vi "Power Measurement Test.vi"(8 "error in (no error)":errorcluster, 9 "Power Measurements":string[](array[string]), 10 "Position":u32, 11 "Measurement in":refnum<class "Measurement.lvclass">) -> (0 "error out":errorcluster, 3 "Passed":bool)   [LabVIEW 2015, in "Measurement.lvclass"]
uses:
  Measurement.lvclass
  Driver Test/Measurement Type -- Enum.ctl
  <vilib>/regexp/Match Regular Expression.xnode
  Driver Test/Driver Test.lvclass
  Test Class/Test Class.lvclass
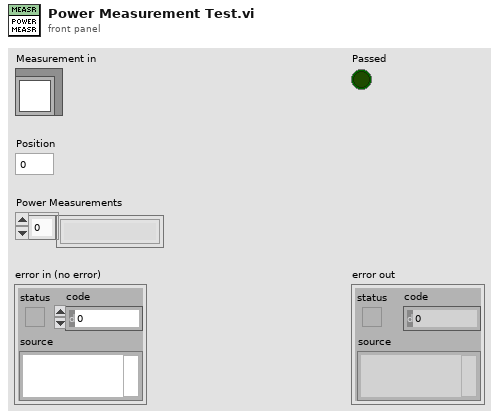
[diagram p1: front panel]
types:
  T1 = typedef "Driver Test.lvclass/Measurement Type -- Enum.ctl" = enum16{"DPM", "DAQmx", "ACPS Voltage", "ACPS Current", "ACPS Power", "DCPS Voltage", "DCPS Current", "DCPS Power"}
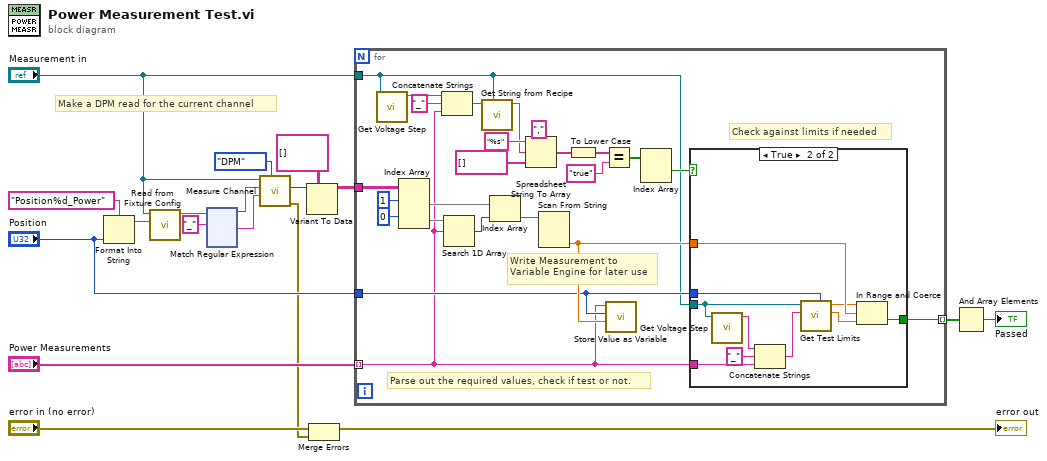
[diagram p0: block diagram]
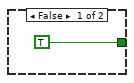
[diagram p2: hidden frame]
diagram:
  # "Make a DPM read for the current channel"
  n1 = Format Into String(format string="Position%d_Power", "Position") -> (resulting string=w16:string)  [unwired: 2 in, 1 out]
  n2 = call-dynamic "Read from Fixture Config.vi"("Key"=w16, "Test Class in"="Measurement in") -> ("Instrument Info"=w13:string)  [unwired: 8 in, 1 out]
  n3 = xnode "Match Regular Expression"("input string"=w13, "regular expression"="_") -> ("before match"=w12:string, "after match"=w11:string)  [unwired: 4 in, 3 out]
  n4 = call "Measure Channel.vi"("Measurement Type"=Measurement_Type_--_Enum."DPM", "Channel"=w11, "Instrument"=w12, "Driver Test in"="Measurement in") -> ("error out"=w3:errorcluster, "Additional Info"=w10:variant)  [unwired: 5 in, 1 out]
  n5 = Variant To Data(type=string[][] [] ("regular expression"), Variant=w10) -> (data=w7:string[][])  [unwired: 1 in, 1 out]
  n6 = Merge Errors("error in (no error)", w3) -> (→"error out":errorcluster)
  n7 = for {
    tunnel: "Power Measurements" -> [w20] mode=indexing
    tunnel: w7 -> [w42]
    tunnel: "Position" -> [w23]
    tunnel: "Measurement in" -> [w21]
    tunnel: [w19] -> w2 mode=indexing
    # "Check against limits if needed"
    # "Write Measurement to \nVariable Engine for later use"
    # "Parse out the required values, check if test or not."
    n8 = call "Get Voltage Step.vi"("Driver Test in"=w21) -> ("Voltage Step"=w28:string)  [unwired: 9 in, 1 out]
    n9 = Index Array(array=w42, index (row) #1=1 ("disabled index (col)"), index (row) #2=0 ("disabled index (col)")) -> (element #1=w38:string[], element #2=w39:string[])  [unwired: 2 in]
    n10 = Concatenate Strings(w28, "_" ("element"), w20) -> (w27:string)
    n11 = Search 1D Array(1D array=w39, element=w20) -> (index of element=w37:i32)  [unwired: 1 in]
    n12 = call "Get String from Recipe.vi"("Test Class in"=w21, "Name"=w27) -> ("Value"=w26:string)  [unwired: 7 in, 2 out]
    n13 = Index Array(array=w38, index=w37) -> (element=w25:string)
    n14 = Spreadsheet String To Array(delimiter (Tab)=",", format string="%s", spreadsheet string=w26, array type (2D Dbl)=string[] []) -> (array=w33:string[])
    n15 = Scan From String(input string=w25) -> (output 1=w24:dbl)  [unwired: 4 in, 3 out]
    n16 = To Lower Case(string=w33) -> (all lower case string=w34:string[])
    n17 = Equal?(x=w34, y="true") -> (x = y?=w36:bool[])
    n18 = call "Store Value as Variable.vi"("Value"=w24, "Position"=w23, "Variable Name"=w20) -> ()  [unwired: 9 in]
    n19 = Index Array(array=w36) -> (element #1=w22:bool)  [unwired: 2 in, 1 out]
    n20 = case shown="True" w22 {
      tunnel: w21 -> [_ w48]
      tunnel: w20 -> [_ w45]
      tunnel: [TRUE w53] -> w19
      tunnel: w24 -> [_ w52]
      tunnel: w23 -> [_ w51]
      frame False {
      }
      frame True {
        n21 = call "Get Voltage Step.vi"("Driver Test in"=w48) -> ("Voltage Step"=w46:string)  [unwired: 9 in, 1 out]
        n22 = Concatenate Strings(w46, "_" ("string"), w45) -> (w44:string)
        n23 = call "Get Test Limits.vi"("Position"=w51, "Channel"=w44, "Test Class in"=w48) -> ("Lower Limit"=w49:dbl, "Upper Limit"=w50:dbl)  [unwired: 6 in, 1 out]
        n24 = In Range and Coerce(upper limit=w50, x=w52, lower limit=w49) -> (In Range?=w53:bool)  [unwired: 1 out]
      }
    }
  }
  n25 = And Array Elements(Boolean array=w2) -> (logical AND=→"Passed":bool)
